vi "未命名 1.vi"(0 "Offset":dbl caption="偏移量", 2 "Reset Signal":bool caption="重置信号", 5 "Frequency":dbl=10.1 caption="频率", 7 "Amplitude":dbl=1.0 caption="幅值", 9 "Phase":dbl caption="相位", 11 "error in (no error)":errorcluster caption="错误输入（无错误）") -> (4 "正弦":dynamicdata(graph), 15 "error out":errorcluster caption="错误输出")   [LabVIEW 2018]
doc: "仿真正弦波、方波、三角波、锯齿波和噪声。\n--------------------\n\n该Express VI配置如下:\n\n信号类型: 正弦\n频率: 10.1 Hz\n幅值: 1\n相位: 0\n偏移量: 0\n采样率: 1000 Hz\n采样数: 100 （自动）\n定时: 以可达到的最快速度运行\n时间标识: 相对"
panel:
  in  "试验":i32=1
  in  "Seed Number":dbl=-1.0 caption="种子值"
  in  "标准差":dbl=0.6
  in  "Duty Cycle (%)":dbl=50.0 caption="占空比(%)"
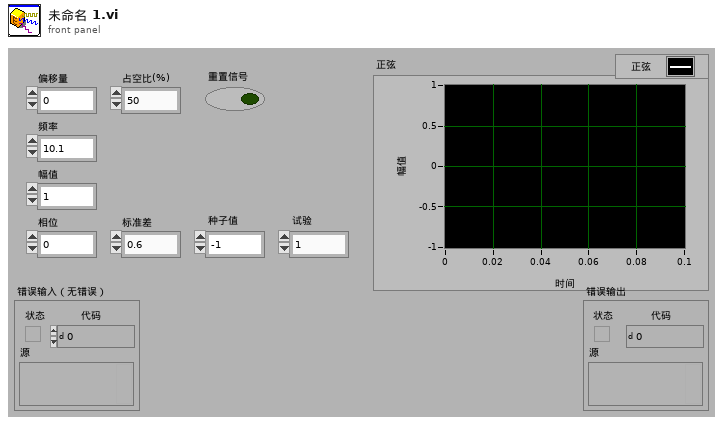
[diagram p1: front panel]
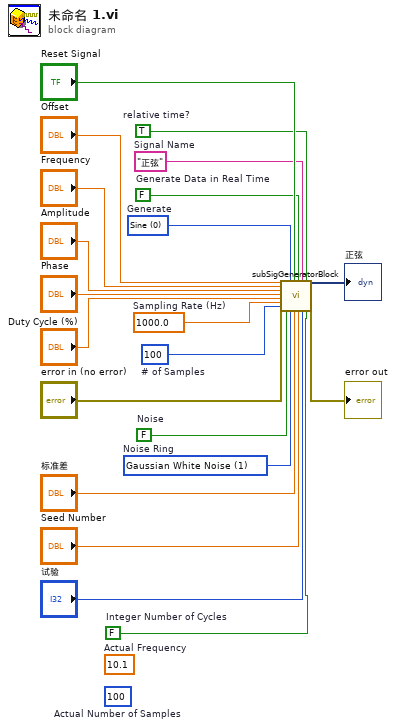
[diagram p0: block diagram]
diagram:
  (unwired) 10.1  # Actual Frequency
  (unwired) 100  # Actual Number of Samples
  w1 = FALSE  # Integer Number of Cycles
  w5 = u16 1 items=["Uniform White Noise", "Gaussian White Noise", "Periodic Random Noise", "Gamma Noise", "Poisson Noise", "Binomial Noise", "Bernoulli Noise", "MLS Sequence "]  # Noise Ring
  w6 = FALSE  # Noise
  w9 = TRUE  # relative time?
  w10 = "正弦"  # Signal Name
  w11 = FALSE  # Generate Data in Real Time
  w13 = u16 0 items=["Sine", "Square", "Triangle", "Sawtooth", "DC"]  # Generate
  w15 = 100  # # of Samples
  w17 = 1000.0  # Sampling Rate (Hz)
  n1 = call <vilib>:"subSigGeneratorBlock.vi"("Offset"="Offset", "Frequency"="Frequency", "Amplitude"="Amplitude", "Phase"="Phase", "Duty Cycle (%)"="Duty Cycle (%)", "Sampling Rate (Hz)"=w17, "# of Samples"=w15, "error in (no error)"="error in (no error)", "Noise"=w6, "Generate"=w13, "Noise Ring"=w5, "Reset Signal"="Reset Signal", "Noise Amplitude"="标准差", "Generate Data in Real Time"=w11, "Seed Number"="Seed Number", "Signal Name"=w10, "trials"="试验", "relative time?"=w9, "Integer Number of Cycles"=w1) -> ("Signal"=→"正弦":dynamicdata, "error out"=→"error out":errorcluster)  [unwired: 7 in]
